vi "Untitled 1.vi"() -> ()   [LabVIEW 2019]
uses:
  <vilib>/Rock Robotics/WPI/Solenoid/WPI_SolenoidValue.ctl
  <vilib>/Rock Robotics/WPI/ThirdParty/Phoenix-LabVIEW/Motor Controller/Controls/CTRE_Phoenix_MotorControl_ControlMode.ctl
  <vilib>/Rock Robotics/WPI/Utilities/WPI_GetSetVariantRefNum.vi
  <vilib>/Rock Robotics/Network Tables/NT Write Number.vi
  <vilib>/Rock Robotics/WPI/Solenoid/WPI_SolenoidSetEnum.vi
panel:
  in  "Output":dbl=0.05
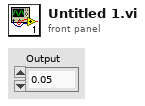
[diagram p1: front panel]
types:
  T1 = typedef "WPI_JoystickDevRef.ctl" = cluster{"Device":T2}
  T2 = typedef "WPI_JoystickDeviceEnum.ctl" = enum16{"USB 0", "USB 1", "USB 2", "USB 3", "USB 4", "USB 5"}
  T3 = typedef "WPI_SolenoidDevRef.ctl" = cluster{"DevStatus":errorcluster, "Pneumatics Control Module":u8, "Forward Solenoid Channel":T4, "Reverse Solenoid Channel":T4}
  T4 = typedef "WPI_SolenoidChannel.ctl" = enum8{"Solenoid 0", "Solenoid 1", "Solenoid 2", "Solenoid 3", "Solenoid 4", "Solenoid 5", "Solenoid 6", "Solenoid 7", "Invalid"}
  T5 = typedef "WPI_MotorControlDeviceRef.ctl" = cluster{"DeviceStatus":errorcluster, "Type":T6, "PWM":cluster{"PWM Channel":T7, "DeadBand":T8}, "CAN":cluster{"Device Number":u8, "SetOutput VI Ref":variant, "GetOutput VI Ref":variant, "Enable VI Ref":variant, "Disable VI Ref":variant, "Data":variant}, "Invert":bool, "DIO PWM":cluster{"PWM \"Enable\" Channel":T7, "DIOChannel":T9, "PWM Rate":dbl}}
  T6 = typedef "WPI_MotorControlType.ctl" = enum16{"PWM", "CAN", "DIO PWM"}
  T7 = typedef "FPGA_DIOPWMChannel.ctl" = enum8{"PWM 0", "PWM 1", "PWM 2", "PWM 3", "PWM 4", "PWM 5", "PWM 6", "PWM 7", "PWM 8", "PWM 9", "PWM MXP 0", "PWM MXP 1", "PWM MXP 2", "PWM MXP 3", "PWM MXP 4", "PWM MXP 5", "PWM MXP 6", "PWM MXP 7", "PWM MXP 8", "PWM MXP 9", "Invalid"}
  T8 = typedef "WPI_PWMDeadband.ctl" = cluster{"Name":string, "maxPositivePwm":i32, "minPositivePwm":i32, "centerPwm":i32, "maxNegativePwm":i32, "minNegativePwm":i32, "angularRange":u16}
  T9 = typedef "FPGA_DIOChannel.ctl" = enum8{"DIO 0", "DIO 1", "DIO 2", "DIO 3", "DIO 4", "DIO 5", "DIO 6", "DIO 7", "DIO 8", "DIO 9", "DIO MXP 0", "DIO MXP 1", "DIO MXP 2", "DIO MXP 3", "DIO MXP 4", "DIO MXP 5", "DIO MXP 6", "DIO MXP 7", "DIO MXP 8", "DIO MXP 9", "DIO MXP 10", "DIO MXP 11", "DIO MXP 12", "DIO MXP 13", "DIO MXP 14", "DIO MXP 15", "SPI Port CS1", "SPI Port CS2", "SPI Port CS3", "SPI Port MISO", "SPI Port MOSI", "Invalid"}
  T10 = typedef "WPI_CompressorDevRef.ctl" = cluster{"DevStatus":errorcluster, "Pneumatics Control Module":u8}
  T11 = typedef "WPI_SolenoidValue.ctl" = enum16{"Off", "On", "Forward", "Reverse"}
  T12 = typedef "CTRE_Phoenix_MotorControl_ControlMode.ctl" = u16
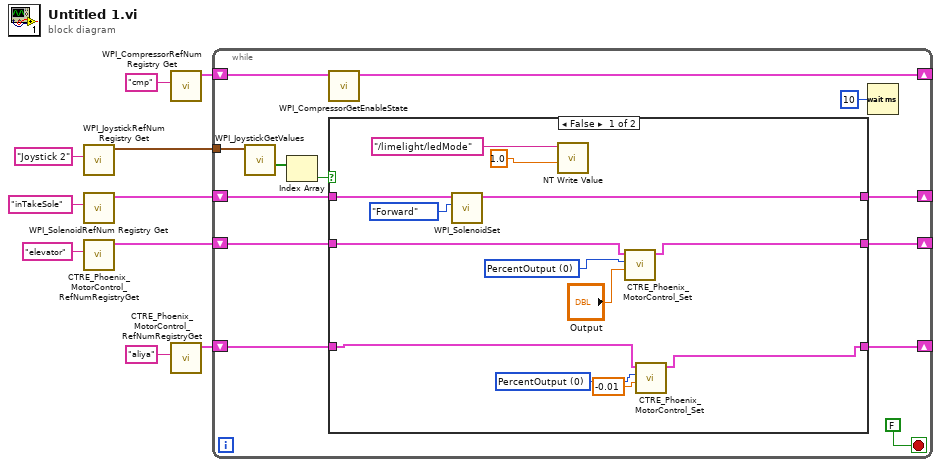
[diagram p0: block diagram]
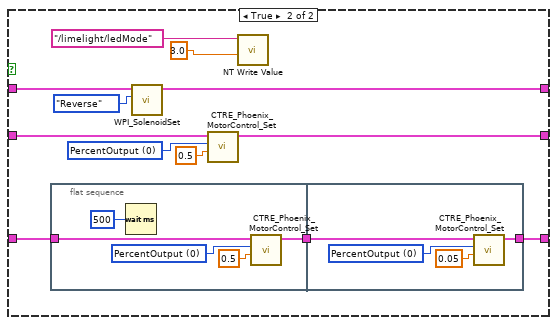
[diagram p2: hidden frame]
diagram:
  n1 = call <vilib>:"WPI_JoystickRefNum Registry Get.vi"("refnum name"="Joystick 2") -> ("JoystickDevRef"=w9:T1)  [unwired: 9 in, 1 out]
  n2 = call <vilib>:"WPI_SolenoidRefNum Registry Get.vi"("refnum name"="inTakeSole") -> ("SolenoidDevRef"=w3:T3)  [unwired: 9 in, 1 out]
  n3 = call <vilib>:"CTRE_Phoenix_MotorControl_RefNumRegistryGet.vi"("refnum name"="elevator") -> ("PhoenixMotorControlDevRef"=w1:T5)  [unwired: 9 in, 1 out]
  n4 = call <vilib>:"WPI_CompressorRefNum Registry Get.vi"("refnum name"="cmp") -> ("CompressorDevRef"=w5:T10)  [unwired: 9 in, 1 out]
  n5 = call <vilib>:"CTRE_Phoenix_MotorControl_RefNumRegistryGet.vi"("refnum name"="aliya") -> ("PhoenixMotorControlDevRef"=w7:T5)  [unwired: 9 in, 1 out]
  n6 = while {
    tunnel: w9 -> [w23]
    shift-right: [w18] -> _
    shift-left: w7 -> [w20]
    shift-right: [w17] -> _
    shift-left: w5 -> [w16]
    shift-right: [w12] -> _
    shift-left: w3 -> [w15]
    shift-right: [w13] -> _
    shift-left: w1 -> [w14]
    stop <- FALSE stop-if-true
    n7 = call <vilib>:"WPI_JoystickGetValues.vi"("JoystickDevRef"=w23) -> ("Buttons"=w22:bool[])  [unwired: 6 in, 4 out]
    n8 = Index Array(array=w22) -> (element=w21:bool)  [unwired: 1 in]
    n9 = call <vilib>:"WPI_CompressorGetEnableState.vi"("CompressorDevRef"=w16) -> ("CompressorDevRef"=w17:T10)  [unwired: 7 in, 3 out]
    n10 = case shown="False" w21 {
      tunnel: w20 -> [w29 w46]
      tunnel: [w28 w45] -> w18
      tunnel: w15 -> [w34 w42]
      tunnel: w14 -> [w26 w41]
      tunnel: [w25 w40] -> w13
      tunnel: [w32 w37] -> w12
      frame False {
        w30 = T12 0 items=["PercentOutput"=0, "Position"=1, "Velocity"=2, "Current"=3, "Follower"=5, "MotionProfile"=6, "MotionMagic"=7, "MotionProfileArc"=10, "Disabled"=15] ("Control Mode")
        w27 = T12 0 items=["PercentOutput"=0, "Position"=1, "Velocity"=2, "Current"=3, "Follower"=5, "MotionProfile"=6, "MotionMagic"=7, "MotionProfileArc"=10, "Disabled"=15] ("Control Mode")
        n11 = call-poly <vilib>:"WPI_SolenoidSet.vi"("Value"=WPI_SolenoidValue."Forward", "SolenoidDevRef"=w34) -> ("SolenoidDevRef"=w32:T3)  [unwired: 8 in, 1 out]
        n12 = call-poly <vilib>:"NT Write Value.vi"("Numeric"=1.0, "Name"="/limelight/ledMode") -> ()  [unwired: 9 in, 1 out]
        n13 = call <vilib>:"CTRE_Phoenix_MotorControl_Set.vi"("Output"="Output", "Control Mode"=w27, "PhoenixMotorControlDevRef"=w26) -> ("PhoenixMotorControlDevRef"=w25:T5)  [unwired: 7 in, 1 out]
        n14 = call <vilib>:"CTRE_Phoenix_MotorControl_Set.vi"("Output"=-0.01, "Control Mode"=w30, "PhoenixMotorControlDevRef"=w29) -> ("PhoenixMotorControlDevRef"=w28:T5)  [unwired: 7 in, 1 out]
      }
      frame True {
        w39 = T12 0 items=["PercentOutput"=0, "Position"=1, "Velocity"=2, "Current"=3, "Follower"=5, "MotionProfile"=6, "MotionMagic"=7, "MotionProfileArc"=10, "Disabled"=15] ("Control Mode")
        n15 = flat-sequence {
          tunnel: w46 -> [w53]
          tunnel: [w49] -> w44
          tunnel: [w56] -> w45
          tunnel: w44 -> [w55]
          frame #0 {
            w52 = T12 0 items=["PercentOutput"=0, "Position"=1, "Velocity"=2, "Current"=3, "Follower"=5, "MotionProfile"=6, "MotionMagic"=7, "MotionProfileArc"=10, "Disabled"=15] ("Control Mode")
            n16 = Wait (ms)(milliseconds to wait=u32 500) -> ()  [unwired: 1 out]
            n17 = call <vilib>:"CTRE_Phoenix_MotorControl_Set.vi"("Output"=0.5, "Control Mode"=w52, "PhoenixMotorControlDevRef"=w53) -> ("PhoenixMotorControlDevRef"=w49:T5)  [unwired: 7 in, 1 out]
          }
          frame #1 {
            w54 = T12 0 items=["PercentOutput"=0, "Position"=1, "Velocity"=2, "Current"=3, "Follower"=5, "MotionProfile"=6, "MotionMagic"=7, "MotionProfileArc"=10, "Disabled"=15] ("Control Mode")
            n18 = call <vilib>:"CTRE_Phoenix_MotorControl_Set.vi"("Output"=0.05, "Control Mode"=w54, "PhoenixMotorControlDevRef"=w55) -> ("PhoenixMotorControlDevRef"=w56:T5)  [unwired: 7 in, 1 out]
          }
        }
        n19 = call-poly <vilib>:"WPI_SolenoidSet.vi"("Value"=WPI_SolenoidValue."Reverse", "SolenoidDevRef"=w42) -> ("SolenoidDevRef"=w37:T3)  [unwired: 8 in, 1 out]
        n20 = call <vilib>:"CTRE_Phoenix_MotorControl_Set.vi"("Output"=0.5, "Control Mode"=w39, "PhoenixMotorControlDevRef"=w41) -> ("PhoenixMotorControlDevRef"=w40:T5)  [unwired: 7 in, 1 out]
        n21 = call-poly <vilib>:"NT Write Value.vi"("Numeric"=3.0, "Name"="/limelight/ledMode") -> ()  [unwired: 9 in, 1 out]
      }
    }
    n22 = Wait (ms)(milliseconds to wait=u32 10) -> ()  [unwired: 1 out]
  }
